vi "Periodic Tasks.vi"(8 "error in":errorcluster) -> ()   [LabVIEW 2019]
doc: "This VI runs in parallel to other tasks. It can contain as many user-defined periodic loops as you need. These can carry out PID or other sorts of timed response."
uses:
  <vilib>/Rock Robotics/WPI/DriverStation/WPI_DriverStationRobotMode2.ctl
  <vilib>/Rock Robotics/WPI/ThirdParty/Phoenix-LabVIEW/Motor Controller/Controls/CTRE_Phoenix_MotorControl_ControlMode.ctl
  <vilib>/Rock Robotics/WPI/Utilities/WPI_GetSetVariantRefNum.vi
  Robot Global Data.vi
  <vilib>/Rock Robotics/WPI/ThirdParty/Phoenix-LabVIEW/Pigeon IMU/CTRE_PigeonIMU_GetYPR.vi
  <vilib>/Rock Robotics/WPI/ThirdParty/Phoenix-LabVIEW/Motor Controller/Get/CTRE_Phoenix_MotorController_GetSelectedSensorData.vi
  <vilib>/Rock Robotics/Network Tables/NT Read Number.vi
  <vilib>/Rock Robotics/Network Tables/NT Write Number.vi
  <vilib>/addons/control/pid/pid.llb/PID (DBL).vi
  <vilib>/ptbypt/NI_PtbyPt.lvlib
  <vilib>/addons/control/pid/NI_PID_pid.lvlib
panel:
  out "Waveform Chart":dbl(graph)
  in  "RPM Range":dbl=120.0
  in  "Intake Speed 2":dbl(slide)=-1.0 min=-1.0 max=1.0 scale=-1.0..1.0
  in  "PID gains Shooter":T1={"proportional gain (Kc)"=0.0008, "integral time (Ti, min)"=0.0, "derivative time (Td, min)"=0.00015} {"derivative time (Td, min)" format="%.6f"; "integral time (Ti, min)" format="%.6f"; "proportional gain (Kc)" format="%.5f"}
  out "RPM Gauge":dbl
  in  "Shooter RPM":dbl=6000.0
  in  "Shooter RPM 3":dbl
  in  "Feeder Speed":dbl(slide)=1.0 min=-1.0 max=1.0 scale=-1.0..1.0
  in  "Conveyer Speed":dbl(slide)=-0.30612244897959184 min=-1.0 max=1.0 scale=-1.0..1.0
  in  "Intake Speed":dbl(slide)=1.0 min=-1.0 max=1.0 scale=-1.0..1.0
  in  "Feeder Speed 3":dbl(slide)=-1.0 min=-1.0 max=1.0 scale=-1.0..1.0
  in  "Conveyer Speed 3":dbl(slide)=0.16326530612244894 min=-1.0 max=1.0 scale=-1.0..1.0
  in  "Intake Speed 3":dbl(slide)=1.0 min=-1.0 max=1.0 scale=-1.0..1.0
  out "Turret Angle":dbl=90.48445184525423
  in  "PID gains Turret":T1={"proportional gain (Kc)"=0.01, "integral time (Ti, min)"=0.0, "derivative time (Td, min)"=0.0} {"derivative time (Td, min)" format="%.5f"; "integral time (Ti, min)" format="%.5f"; "proportional gain (Kc)" format="%.5f"}
  out "Go Slow?":bool
  in  "Z-axis rate modifier":dbl=0.7 format="%#_13g"
  in  "Slow Drive Speed %":dbl=0.75
  out "Robot Centric?":bool
  out "Sensor Loop Speed":u32=23
  in  "Sensor wait":u32=25
  out "Gyro Yaw Out":dbl=-111.95 format="%#_13g"
  out "Drive Loop Speed":u32=24
  in  "Drive wait":u32=25
  in  "Rot Pt Y":dbl format="%#_13g"
  in  "Rot Pt X":dbl format="%#_13g"
  out "Joystick Loop Speed":u32=24
  in  "Joystick wait":u32=25
  # "Intake"
  # "Shooter"
  # "Spinny wheel thing"
  # ".00050\n.000000\n.000100"
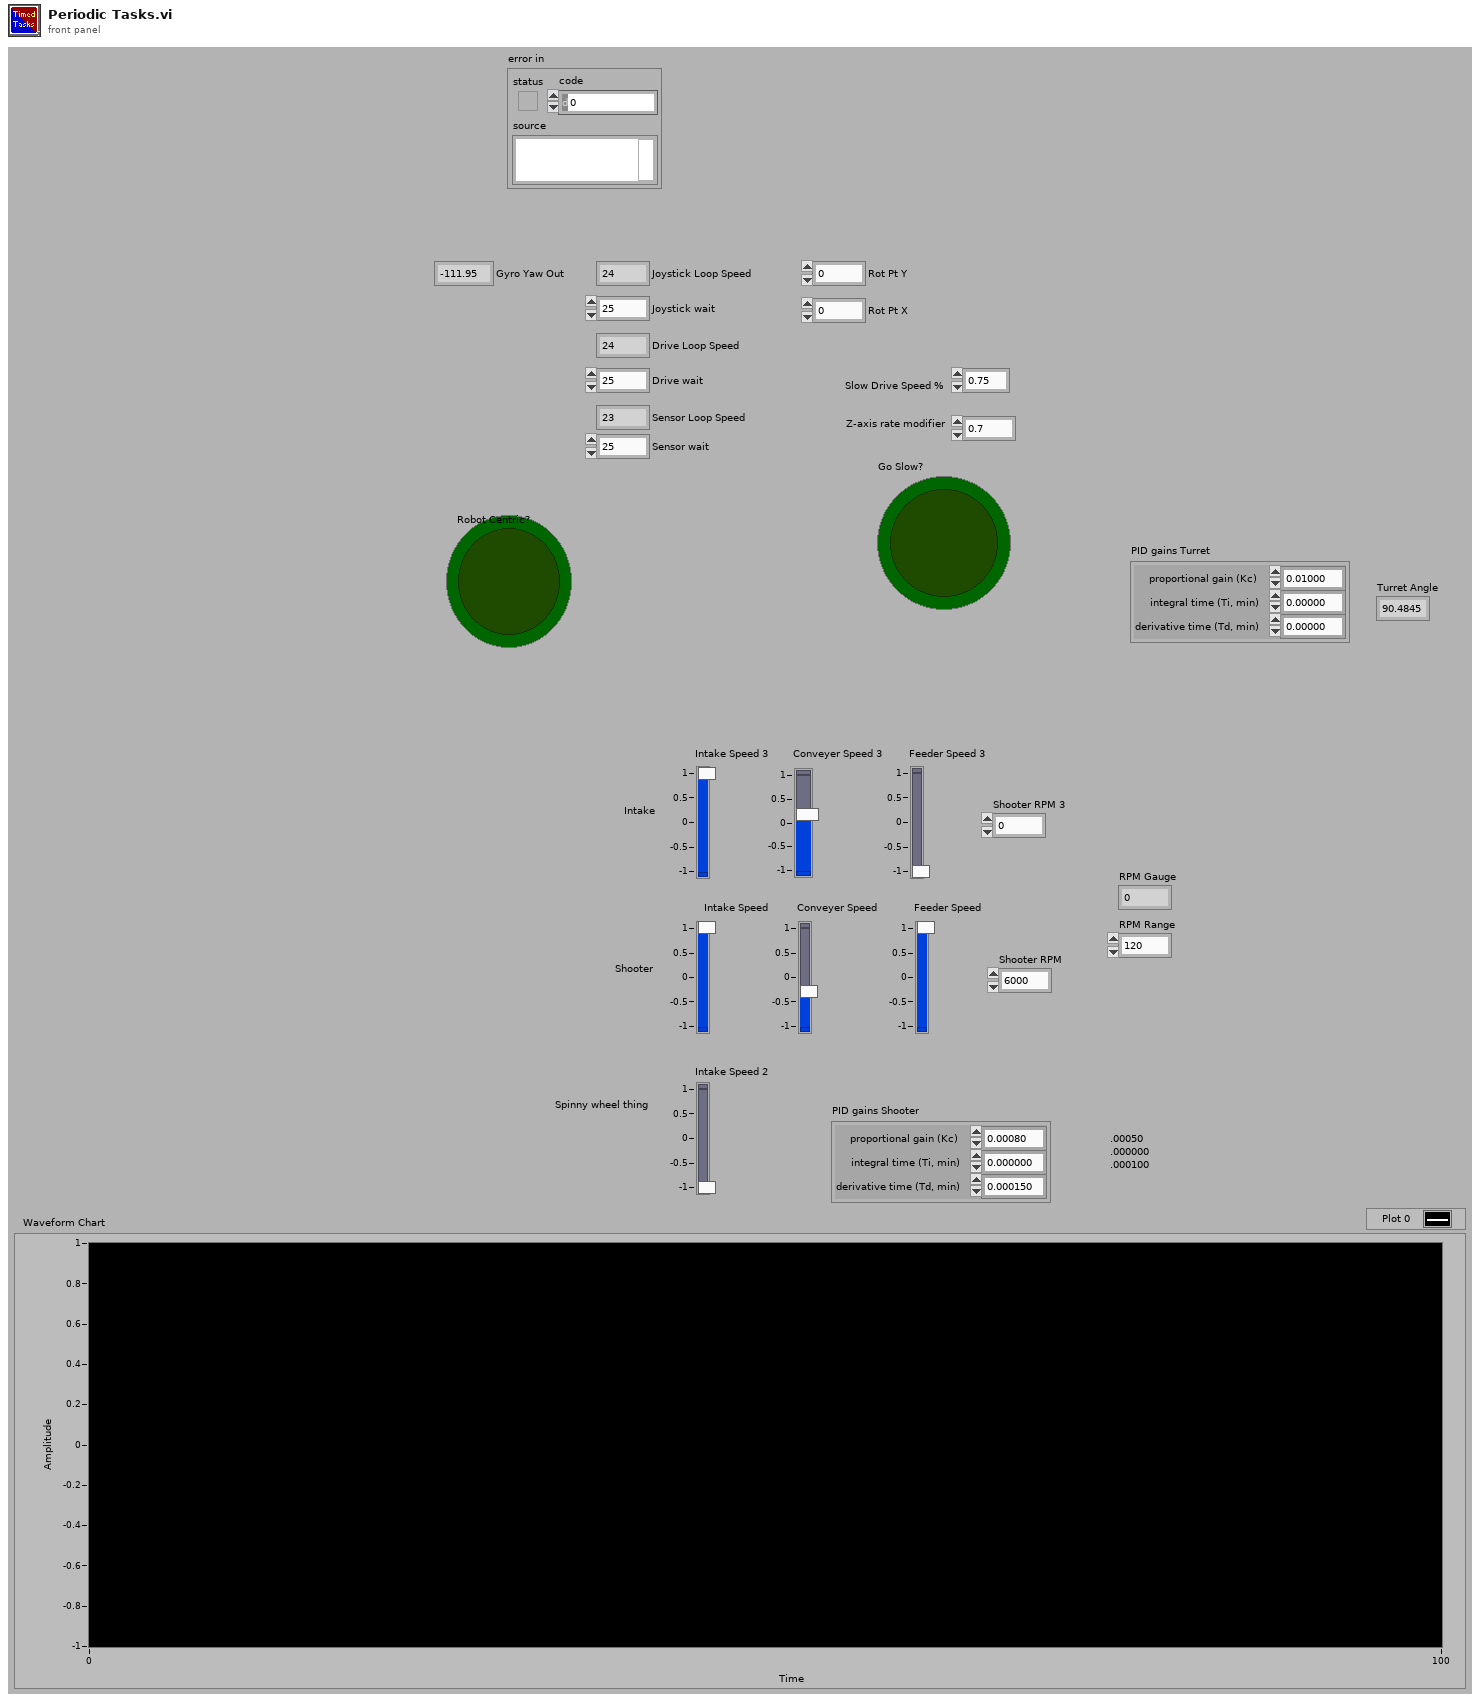
[diagram p1: front panel]
types:
  T1 = cluster{"proportional gain (Kc)":dbl, "integral time (Ti, min)":dbl, "derivative time (Td, min)":dbl}
  T2 = typedef "WPI_JoystickDevRef.ctl" = cluster{"Device":T3}
  T3 = typedef "WPI_JoystickDeviceEnum.ctl" = enum16{"USB 0", "USB 1", "USB 2", "USB 3", "USB 4", "USB 5"}
  T4 = typedef "WPI_DriverStationRobotMode2.ctl" = enum16{"Autonomous Disabled", "Autonomous Enabled", "Teleop Disabled", "Teleop Enabled", "Disconnected", "Finish", "Test Disabled", "Test Enabled", "Emergency Stopped"}
  T5 = typedef "CTRE_Phoenix_MotorControl_ControlMode.ctl" = u16
  T6 = typedef "CTRE_PigeonIMU_DeviceRef.ctl" = cluster{"DeviceStatus":errorcluster, "Device Number":u8, "Type":T7, "Device ID":u32, "Handle":u64, "UsageFrame":u32, "Library Path":path}
  T7 = typedef "CTRE_PigeonIMU_ConnectionType.ctl" = u32
  T8 = typedef "WPI_ServoDeviceRef.ctl" = cluster{"DeviceStatus":errorcluster, "PWM Channel":T9, "DeadBand":T10}
  T9 = typedef "FPGA_DIOPWMChannel.ctl" = enum8{"PWM 0", "PWM 1", "PWM 2", "PWM 3", "PWM 4", "PWM 5", "PWM 6", "PWM 7", "PWM 8", "PWM 9", "PWM MXP 0", "PWM MXP 1", "PWM MXP 2", "PWM MXP 3", "PWM MXP 4", "PWM MXP 5", "PWM MXP 6", "PWM MXP 7", "PWM MXP 8", "PWM MXP 9", "Invalid"}
  T10 = typedef "WPI_PWMDeadband.ctl" = cluster{"Name":string, "maxPositivePwm":i32, "minPositivePwm":i32, "centerPwm":i32, "maxNegativePwm":i32, "minNegativePwm":i32, "angularRange":u16}
  T11 = typedef "WPI_MotorControlDeviceRef.ctl" = cluster{"DeviceStatus":errorcluster, "Type":T12, "PWM":cluster{"PWM Channel":T9, "DeadBand":T10}, "CAN":cluster{"Device Number":u8, "SetOutput VI Ref":variant, "GetOutput VI Ref":variant, "Enable VI Ref":variant, "Disable VI Ref":variant, "Data":variant}, "Invert":bool, "DIO PWM":cluster{"PWM \"Enable\" Channel":T9, "DIOChannel":T13, "PWM Rate":dbl}}
  T12 = typedef "WPI_MotorControlType.ctl" = enum16{"PWM", "CAN", "DIO PWM"}
  T13 = typedef "FPGA_DIOChannel.ctl" = enum8{"DIO 0", "DIO 1", "DIO 2", "DIO 3", "DIO 4", "DIO 5", "DIO 6", "DIO 7", "DIO 8", "DIO 9", "DIO MXP 0", "DIO MXP 1", "DIO MXP 2", "DIO MXP 3", "DIO MXP 4", "DIO MXP 5", "DIO MXP 6", "DIO MXP 7", "DIO MXP 8", "DIO MXP 9", "DIO MXP 10", "DIO MXP 11", "DIO MXP 12", "DIO MXP 13", "DIO MXP 14", "DIO MXP 15", "SPI Port CS1", "SPI Port CS2", "SPI Port CS3", "SPI Port MISO", "SPI Port MOSI", "Invalid"}
  T14 = cluster{"Rollover":dbl, "Yaw":dbl, "Cont Yaw":dbl}
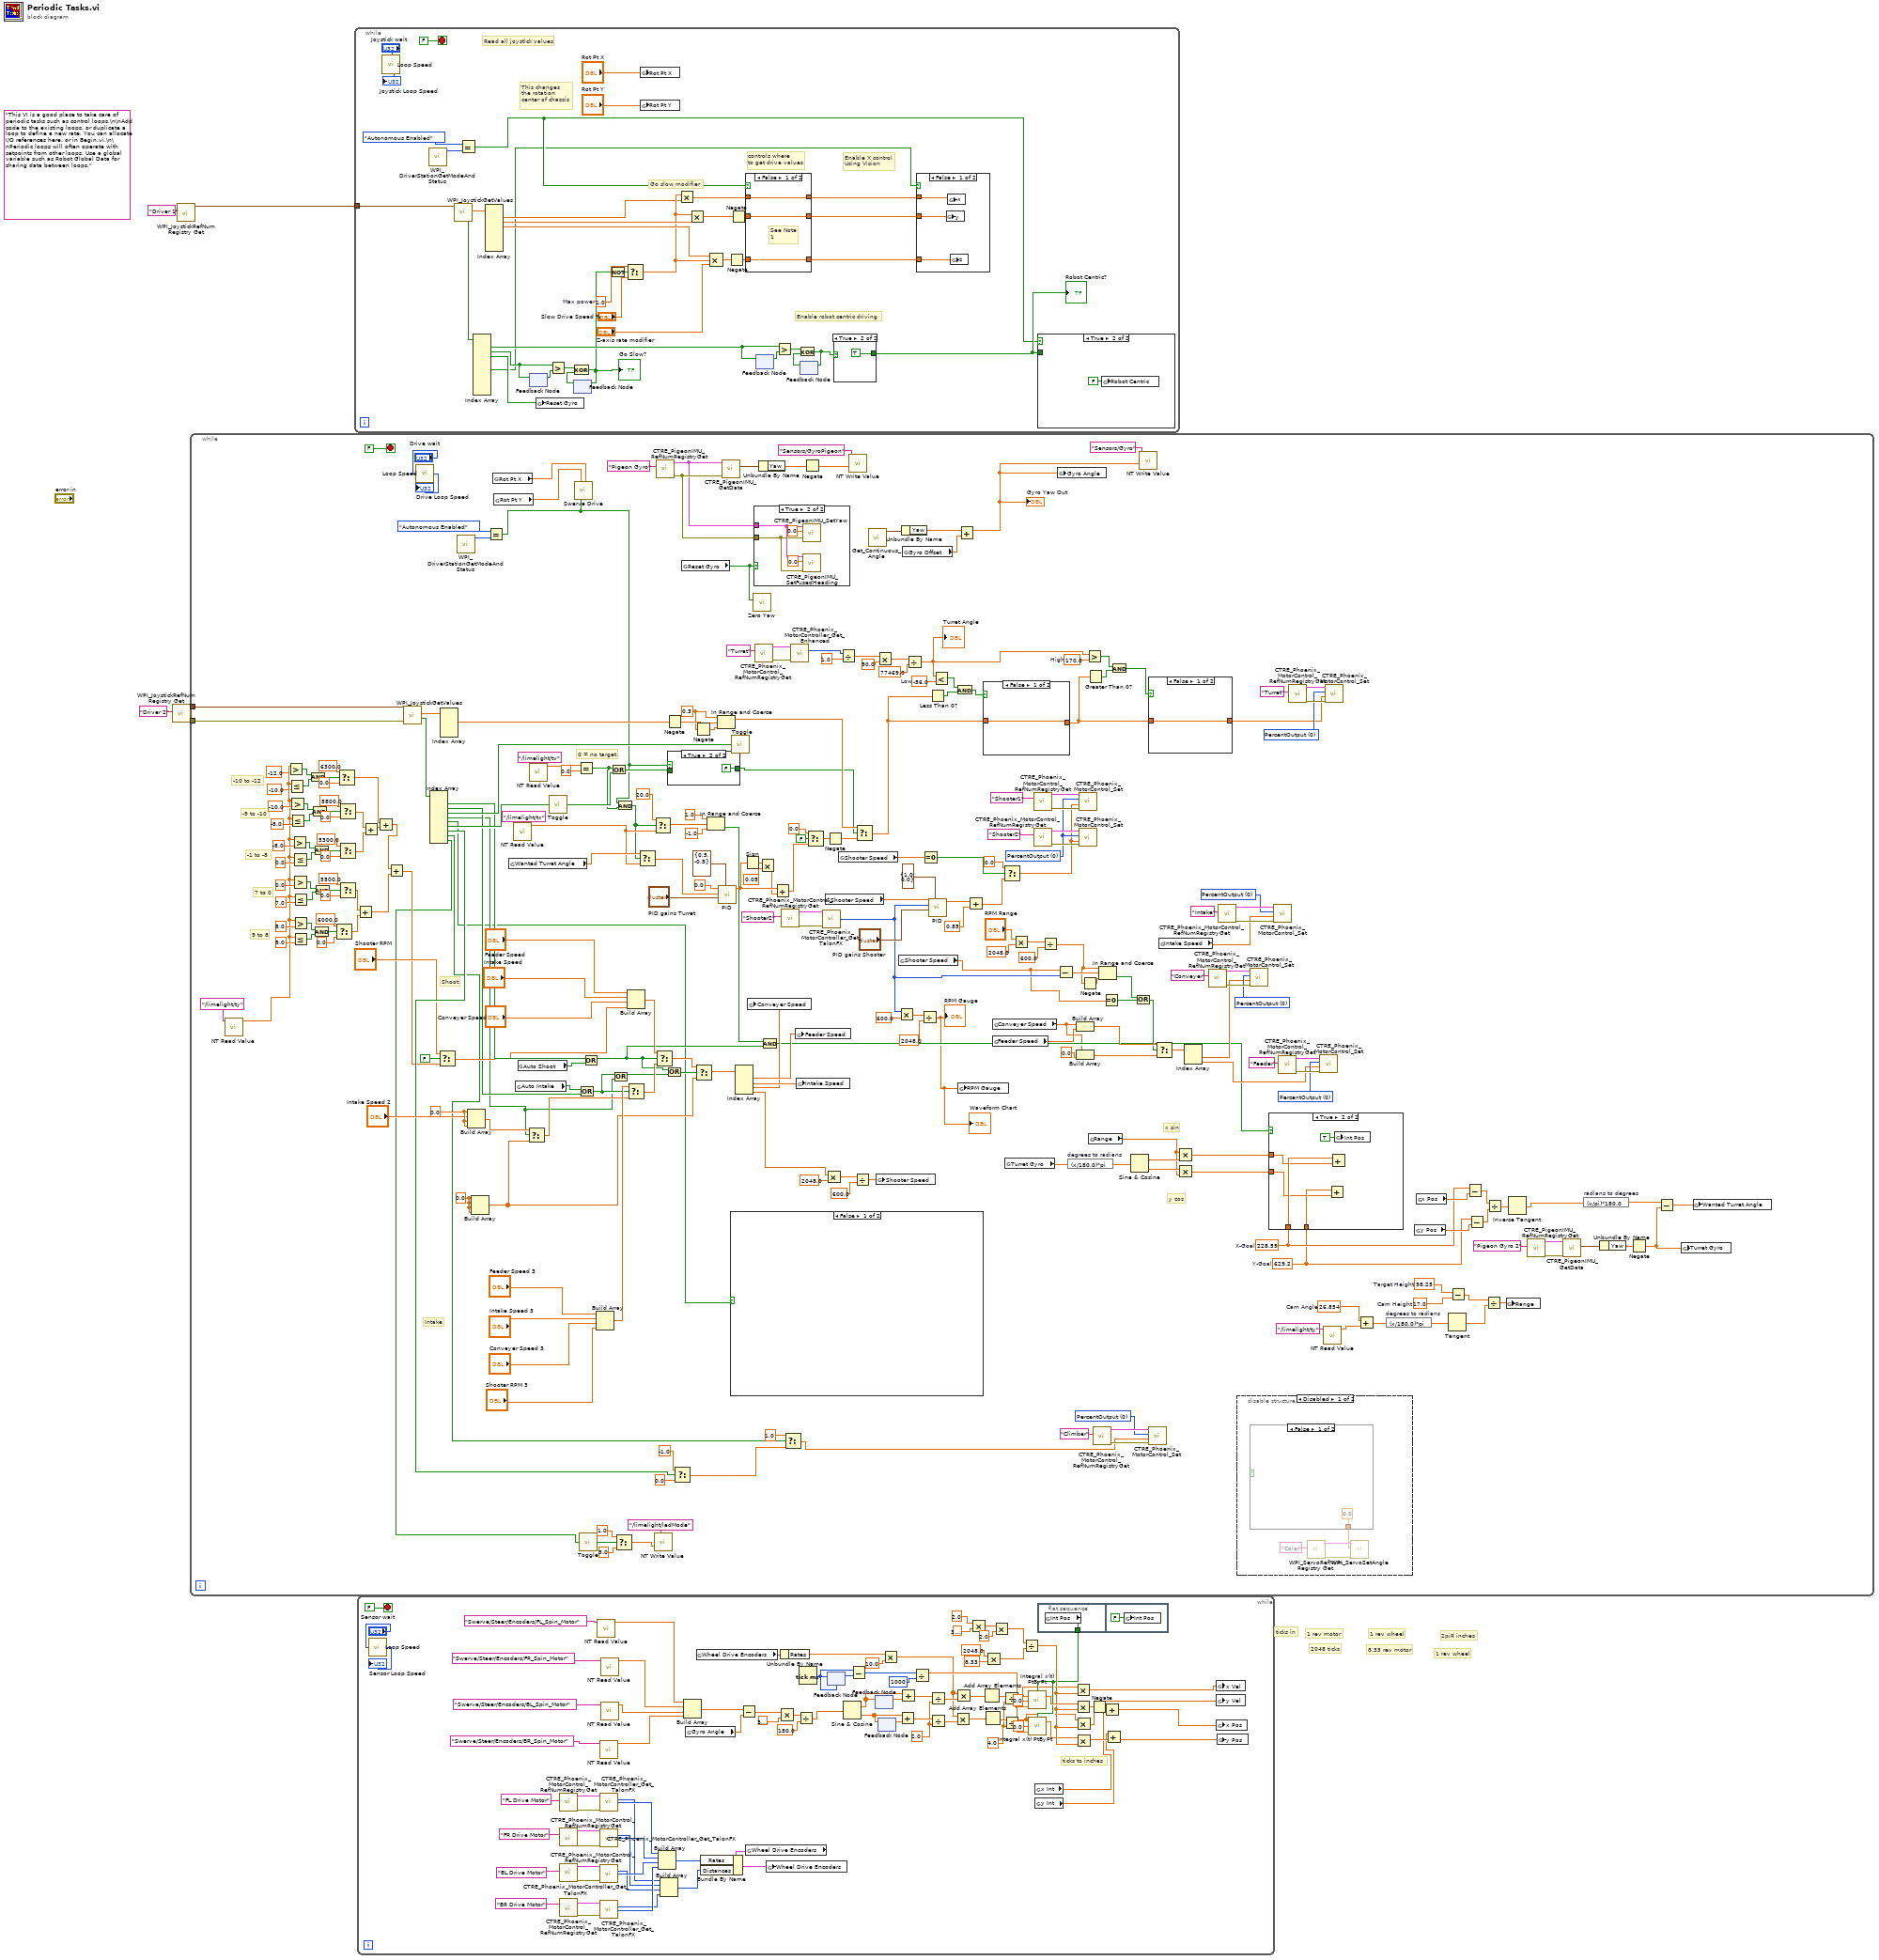
[diagram p0: block diagram]
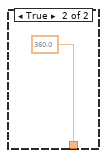
[diagram p2: hidden frame]
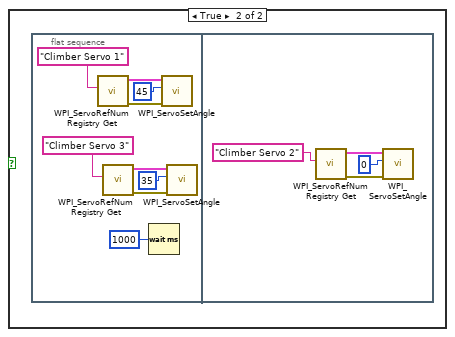
[diagram p6: hidden frame]
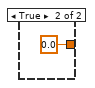
[diagram p7: hidden frame]
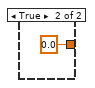
[diagram p8: hidden frame]
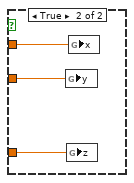
[diagram p10: hidden frame]
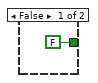
[diagram p11: hidden frame]
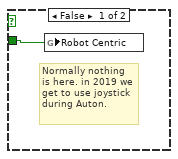
[diagram p12: hidden frame]
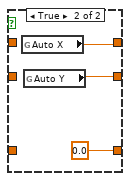
[diagram p13: hidden frame]
diagram:
  (unwired) "This VI is a good place to take care of periodic tasks such as control loops.\n\nAdd code to the existing loops, or duplicate a loop to define a new rate. You can allocate I/O references here, or in Begin.vi.\n\nPeriodic loops will often operate with setpoints from other loops. Use a global variable such as Robot Global Data for sharing data between loops."
  # "2piR inches"
  # "1 rev wheel"
  # "1 rev wheel"
  # "8.33 rev motor"
  # "1 rev motor"
  # "2048 ticks"
  # "ticks in"
  n1 = call <vilib>:"WPI_JoystickRefNum Registry Get.vi"("refnum name"="Driver 2") -> ("error out"=w2:errorcluster, "JoystickDevRef"=w1:T2)  [unwired: 9 in]
  n2 = call <vilib>:"WPI_JoystickRefNum Registry Get.vi"("refnum name"="Driver 1") -> ("JoystickDevRef"=w4:T2)  [unwired: 9 in, 1 out]
  n3 = while {
    tunnel: w2 -> [w233]
    tunnel: w1 -> [w232]
    stop <- FALSE stop-if-true
    w28 = T5 0 items=["PercentOutput"=0, "Position"=1, "Velocity"=2, "Current"=3, "Follower"=5, "MotionProfile"=6, "MotionMagic"=7, "MotionProfileArc"=10, "Disabled"=15] ("Control Mode")
    w109 = 26.854  # Cam Angle
    w112 = 17.0  # Cam Height
    w111 = 98.25  # Target Height
    w116 = 0.3 ("upper limit")
    w145 = T5 0 items=["PercentOutput"=0, "Position"=1, "Velocity"=2, "Current"=3, "Follower"=5, "MotionProfile"=6, "MotionMagic"=7, "MotionProfileArc"=10, "Disabled"=15] ("Control Mode")
    w149 = 228.59  # X-Goal
    w148 = 629.2  # Y-Goal
    w164 = 0.0 ("element")
    w203 = 0.0 ("element")
    w225 = T5 0 items=["PercentOutput"=0, "Position"=1, "Velocity"=2, "Current"=3, "Follower"=5, "MotionProfile"=6, "MotionMagic"=7, "MotionProfileArc"=10, "Disabled"=15] ("Control Mode")
    w223 = T5 0 items=["PercentOutput"=0, "Position"=1, "Velocity"=2, "Current"=3, "Follower"=5, "MotionProfile"=6, "MotionMagic"=7, "MotionProfileArc"=10, "Disabled"=15] ("Control Mode")
    w221 = T5 0 items=["PercentOutput"=0, "Position"=1, "Velocity"=2, "Current"=3, "Follower"=5, "MotionProfile"=6, "MotionMagic"=7, "MotionProfileArc"=10, "Disabled"=15] ("Control Mode")
    w251 = T5 0 items=["PercentOutput"=0, "Position"=1, "Velocity"=2, "Current"=3, "Follower"=5, "MotionProfile"=6, "MotionMagic"=7, "MotionProfileArc"=10, "Disabled"=15] ("Control Mode")
    w255 = 170.0  # High
    w263 = -56.0  # Low
    # "-10 to -12"
    # "-9 to -10"
    # "-1 to -8"
    # "7 to 0"
    # "9 to 8"
    # "y cos"
    # "x sin"
    # "0 = no target"
    # "Intake"
    # "Shoot"
    n4 = call-poly <vilib>:"NT Read Value.vi"("Name"="/limelight/ty") -> ("Numeric"=w8:dbl)  [unwired: 9 in, 1 out]
    n5 = Greater?(x=w8, y=-12.0) -> (0:w16:bool)
    n6 = Less Or Equal?(x=w8, y=-10.0) -> (x <= y?=w15:bool)
    n7 = Greater?(x=w8, y=-10.0) -> (0:w81:bool)
    n8 = Less Or Equal?(x=w8, y=-8.0) -> (x <= y?=w80:bool)
    n9 = Greater?(x=w8, y=-8.0) -> (0:w85:bool)
    n10 = Less Or Equal?(x=w8, y=0.0) -> (x <= y?=w84:bool)
    n11 = Greater?(x=w8, y=0.0) -> (0:w89:bool)
    n12 = Less Or Equal?(x=w8, y=7.0) -> (x <= y?=w88:bool)
    n13 = Greater?(x=w8, y=8.0) -> (0:w90:bool)
    n14 = Less Or Equal?(x=w8, y=9.0) -> (x <= y?=w91:bool)
    n15 = And(x=w16, y=w15) -> (x .and. y?=w14:bool)
    n16 = And(x=w81, y=w80) -> (x .and. y?=w79:bool)
    n17 = And(x=w85, y=w84) -> (x .and. y?=w78:bool)
    n18 = And(x=w90, y=w91) -> (x .and. y?=w76:bool)
    n19 = And(x=w89, y=w88) -> (x .and. y?=w77:bool)
    n20 = Select(t=6000.0, s=w76, f=0.0) -> (s? t:f=w66:dbl)
    n21 = Select(t=6300.0, s=w14, f=0.0) -> (s? t:f=w9:dbl)
    n22 = Select(t=5800.0, s=w79, f=0.0) -> (s? t:f=w65:dbl)
    n23 = Select(t=5300.0, s=w78, f=0.0) -> (s? t:f=w64:dbl)
    n24 = Select(t=5500.0, s=w77, f=0.0) -> (s? t:f=w67:dbl)
    n25 = Add(x=w67, y=w66) -> (x+y=w63:dbl)
    n26 = Add(x=w65, y=w64) -> (x+y=w11:dbl)
    n27 = Add(x=w9, y=w11) -> (x+y=w10:dbl)
    n28 = Add(x=w10, y=w63) -> (x+y=w62:dbl)
    n29 = call <vilib>:"WPI_JoystickGetValues.vi"("error in (no error)"=w233, "JoystickDevRef"=w232) -> ("Buttons"=w202:bool[], "Axes"=w249:dbl[])  [unwired: 5 in, 3 out]
    n30 = call "Loop Speed.vi"("milliseconds to wait"="Drive wait") -> ("Loop Speed"=→"Drive Loop Speed":u32)
    n31 = Index Array(array=w202) -> (element #1=w139:bool, element #2=w114:bool, element #3=w201:bool, element #4=w44:bool, element #5=w26:bool, element #6=w150:bool, element #7=w141:bool, element #8=w53:bool, element #9=w18:bool)  [unwired: 9 in]
    n32 = Select(t="Shooter RPM", s=FALSE, f=w62) -> (s? t:f=w124:dbl)
    n33 = Index Array(array=w249) -> (element #1=w241:dbl)  [unwired: 4 in, 3 out]
    n34 = call <vilib>:"WPI_DriverStationGetModeAndStatus.vi"() -> ("Robot Mode"=w283:T4)  [unwired: 10 in, 1 out]
    n35 = Build Array(w164, "Intake Speed 2", w164, w164) -> (w165:dbl[])
    n36 = Build Array(w203, w203, w203, w203) -> (w166:dbl[])
    n37 = Equal?(x=WPI_DriverStationRobotMode2."Autonomous Enabled", y=w283) -> (x = y?=w57:bool)
    n38 = global read "Robot Global Data.vi" "Rot Pt X"() -> (w274:dbl)
    n39 = global read "Robot Global Data.vi" "Rot Pt Y"() -> (w275:dbl)
    n40 = global read "Robot Global Data.vi" "Wanted Turret Angle"() -> (w152:dbl)
    n41 = call-poly <vilib>:"NT Read Value.vi"("Name"="/limelight/tx") -> ("Numeric"=w133:dbl)  [unwired: 9 in, 1 out]
    n42 = global read "Robot Global Data.vi" "Auto Intake"() -> (w113:bool)
    n43 = global read "Robot Global Data.vi" "Auto Shoot"() -> (w120:bool)
    n44 = Select(t=w165, s=w44, f=w166) -> (s? t:f=w167:dbl[])
    n45 = call-poly <vilib>:"NT Read Value.vi"("Name"="/limelight/tv") -> ("Numeric"=w238:dbl)  [unwired: 9 in, 1 out]
    n46 = call "Toggle.vi"("Input"=w150) -> ("Output"=w151:bool)
    n47 = call "Swerve Drive.vi"("Rot. Point X"=w274, "Auto Controls"=w57, "Rot. Point Y"=w275) -> ()  [unwired: 9 in]
    n48 = Equal?(x=w238, y=0.0) -> (x = y?=w60:bool)
    n49 = Or(x=w113, y=w114) -> (x .or. y?=w115:bool)
    n50 = call "Toggle.vi"("Input"=w18) -> ("Output"=w23:bool)
    n51 = Or(x=w139, y=w120) -> (x .or. y?=w121:bool)
    n52 = Build Array("Feeder Speed 3", "Intake Speed 3", "Conveyer Speed 3", "Shooter RPM 3") -> (w208:dbl[])
    n53 = Or(x=w60, y=w151) -> (x .or. y?=w59:bool)
    n54 = Or(x=w115, y=w44) -> (x .or. y?=w45:bool)
    n55 = Select(t=1.0, s=w23, f=3.0) -> (s? t:f=w19:dbl)
    n56 = And(x=w57, y=w60) -> (x .and. y?=w61:bool)
    n57 = Build Array("Feeder Speed", "Intake Speed", "Conveyer Speed", w124) -> (w212:dbl[])
    n58 = Select(t=w208, s=w115, f=w167) -> (s? t:f=w218:dbl[])
    n59 = Select(t=w152, s=w61, f=w133) -> (s? t:f=w159:dbl)
    n60 = Select(t=20.0, s=w61, f=w133) -> (s? t:f=w135:dbl)
    n61 = call-poly <vilib>:"NT Write Value.vi"("Numeric"=w19, "Name"="/limelight/ledMode") -> ()  [unwired: 9 in, 1 out]
    n62 = Select(t=w212, s=w121, f=w218) -> (s? t:f=w217:dbl[])
    n63 = call <vilib>:"CTRE_PigeonIMU_RefNumRegistryGet.vi"("refnum name"="Pigeon Gyro") -> ("error out"=w280:errorcluster, "PigeonIMUDevRef"=w279:T6)  [unwired: 9 in]
    n64 = Negate(x=w241) -> (-x=w119:dbl)
    n65 = Or(x=w121, y=w45) -> (x .or. y?=w216:bool)
    n66 = case shown="True" w57 {
      tunnel: w59 -> [w291 _]
      tunnel: [w291 FALSE] -> w58
      frame False {
      }
      frame True {
      }
    }
    n67 = Select(t=-1.0, s=w141, f=0.0) -> (s? t:f=w55:dbl)
    n68 = global read "Robot Global Data.vi" "Reset Gyro"() -> (w35:bool)
    n69 = Negate(x=w116) -> (-x=w117:dbl)
    n70 = Select(t=w217, s=w216, f=w166) -> (s? t:f=w207:dbl[])
    n71 = In Range and Coerce(upper limit=1.0, x=w135, lower limit=-1.0) -> (In Range?=w138:bool)  [unwired: 1 out]
    n72 = In Range and Coerce(upper limit=w116, x=w119, lower limit=w117) -> (coerced(x)=w118:dbl)  [unwired: 1 out]
    n73 = call-poly <vilib>:"PID.vi"("output range"=cluster{"output high":dbl, "output low":dbl} {"output high"=0.5, "output low"=-0.5}, "PID gains"="PID gains Turret", "process variable"=w159, "setpoint"=0.0) -> ("output"=w47:dbl)  [unwired: 6 in, 1 out]
    n74 = call-poly <vilib>:"CTRE_PigeonIMU_GetData.vi"("error in (no error)"=w280, "PigeonIMUDevRef"=w279) -> ("Yaw Pitch Roll"=w278:cluster{"Yaw":dbl, "Pitch":dbl, "Roll":dbl})  [unwired: 7 in, 2 out]
    n75 = case shown="False" w26 {
      frame False {
      }
      frame True {
        n76 = flat-sequence {
          frame #0 {
            n77 = call <vilib>:"WPI_ServoRefNum Registry Get.vi"("refnum name"="Climber Servo 1") -> ("error out"=w305:errorcluster, "ServoDeviceRef"=w304:T8)  [unwired: 9 in]
            n78 = call <vilib>:"WPI_ServoRefNum Registry Get.vi"("refnum name"="Climber Servo 3") -> ("error out"=w301:errorcluster, "ServoDeviceRef"=w300:T8)  [unwired: 9 in]
            n79 = Wait (ms)(milliseconds to wait=u32 1000) -> ()  [unwired: 1 out]
            n80 = call <vilib>:"WPI_ServoSetAngle.vi"("error in (no error)"=w305, "Angle"=45, "ServoDeviceRef"=w304) -> ()  [unwired: 7 in, 2 out]
            n81 = call <vilib>:"WPI_ServoSetAngle.vi"("error in (no error)"=w301, "Angle"=35, "ServoDeviceRef"=w300) -> ()  [unwired: 7 in, 2 out]
          }
          frame #1 {
            n82 = call <vilib>:"WPI_ServoRefNum Registry Get.vi"("refnum name"="Climber Servo 2") -> ("error out"=w310:errorcluster, "ServoDeviceRef"=w309:T8)  [unwired: 9 in]
            n83 = call <vilib>:"WPI_ServoSetAngle.vi"("error in (no error)"=w310, "Angle"=0, "ServoDeviceRef"=w309) -> ()  [unwired: 7 in, 2 out]
          }
        }
      }
    }
    n84 = call "Toggle.vi"("Input"=w201) -> ()  [unwired: 1 out]
    n85 = Index Array(array=w207) -> (element #1=w206:dbl, element #2=w205:dbl, element #3=w204:dbl, element #4=w172:dbl)  [unwired: 4 in]
    n86 = Sign(1:w47) -> (0:w49:dbl)
    n87 = global write "Robot Global Data.vi" "Conveyer Speed"(w204) -> ()
    n88 = call <vilib>:"Zero Yaw.vi"("Zero"=w35) -> ()  [unwired: 11 in]
    n89 = case shown="True" w35 {
      tunnel: w279 -> [_ w316]
      tunnel: w280 -> [_ w315]
      frame False {
      }
      frame True {
        n90 = call <vilib>:"CTRE_PigeonIMU_SetYaw.vi"("error in (no error)"=w315, "Value"=0.0, "PigeonIMUDevRef"=w316) -> ()  [unwired: 7 in, 2 out]
        n91 = call <vilib>:"CTRE_PigeonIMU_SetFusedHeading.vi"("error in (no error)"=w315, "Value"=0.0, "PigeonIMUDevRef 2"=w316) -> ()  [unwired: 7 in, 2 out]
      }
    }
    n92 = call <vilib>:"CTRE_Phoenix_MotorControl_RefNumRegistryGet.vi"("refnum name"="Turret") -> ("error out"=w264:errorcluster, "PhoenixMotorControlDevRef"=w265:T11)  [unwired: 9 in]
    n93 = Unbundle By Name(w278) -> ("Yaw"=w281:dbl)
    n94 = Multiply(x=w49, y=0.05) -> (x*y=w46:dbl)
    n95 = And(x=w138, y=w121) -> (x .and. y?=w140:bool)
    n96 = Add(x=w47, y=w46) -> (x+y=w50:dbl)
    n97 = call <vilib>:"CTRE_Phoenix_MotorControl_RefNumRegistryGet.vi"("refnum name"="Shooter2") -> ("error out"=w199:errorcluster, "PhoenixMotorControlDevRef"=w198:T11)  [unwired: 9 in]
    n98 = Select(t=1.0, s=w53, f=w55) -> (s? t:f=w56:dbl)
    n99 = call-poly <vilib>:"CTRE_Phoenix_MotorController_Get_Enhanced.vi"("PhoenixMotorControlDevRef"=w265, "error in"=w264) -> ("Position (Raw Sensor Units)"=w236:i32)  [unwired: 10 in, 3 out]
    n100 = global write "Robot Global Data.vi" "Feeder Speed"(w206) -> ()
    n101 = global write "Robot Global Data.vi" "Intake Speed"(w205) -> ()
    n102 = Negate(x=w281) -> (-x=w36:dbl)
    n103 = Select(t=0.0, s=FALSE, f=w50) -> (s? t:f=w234:dbl)
    n104 = call-poly <vilib>:"CTRE_Phoenix_MotorController_Get_TalonFX.vi"("PhoenixMotorControlDevRef"=w198, "error in"=w199) -> ("Velocity (Raw Sensor Units per 100 ms)"=w132:i32)  [unwired: 10 in, 3 out]
    n105 = global read "Robot Global Data.vi" "Shooter Speed"() -> (w182:dbl)
    n106 = Multiply(x=w172, y=2048.0) -> (x*y=w174:dbl)
    n107 = Negate(x=w234) -> (-x=w137:dbl)
    n108 = global read "Robot Global Data.vi" "Shooter Speed"() -> (w185:dbl)
    n109 = Divide(x=w236, y=1.0) -> (x/y=w270:dbl)
    n110 = call-poly <vilib>:"NT Write Value.vi"("Numeric"=w36, "Name"="Sensors/GyroPigeon") -> ()  [unwired: 9 in, 1 out]
    n111 = Divide(x=w174, y=600.0) -> (x/y=w171:dbl)
    n112 = Select(t=w118, s=w58, f=w137) -> (s? t:f=w240:dbl)
    n113 = call <vilib>:"Get_Continuous_Angle.vi"() -> ("Continuous Angle"=w39:T14)  [unwired: 11 in]
    n114 = Multiply(x=w270, y=90.0) -> (x*y=w268:dbl)
    n115 = global write "Robot Global Data.vi" "Shooter Speed"(w171) -> ()
    n116 = Multiply(x=w132, y=600.0) -> (x*y=w169:dbl)
    n117 = global read "Robot Global Data.vi" "Shooter Speed"() -> (w131:dbl)
    n118 = Unbundle By Name(w39) -> ("Yaw"=w38:dbl)
    n119 = global read "Robot Global Data.vi" "Gyro Offset"() -> (w24:dbl)
    n120 = Divide(x=w268, y=77469.0) -> (x/y=w235:dbl)
    "Turret Angle" <- w235
    n121 = Divide(x=w169, y=2048.0) -> (x/y=w17:dbl)
    "RPM Gauge" <- w17
    "Waveform Chart" <- w17
    n122 = Equal To 0?(x=w185) -> (x = 0?=w183:bool)
    n123 = call-poly <vilib>:"PID.vi"("output range"=cluster{"output high":dbl, "output low":dbl} {"output high"=1.0, "output low"=0.0}, "PID gains"="PID gains Shooter", "process variable"=w132, "setpoint"=w182) -> ("output"=w178:dbl)  [unwired: 6 in, 1 out]
    n124 = Less Than 0?(x=w240) -> (x < 0?=w261:bool)
    n125 = Less?(x=w235, y=w263) -> (x < y?=w262:bool)
    n126 = And(x=w262, y=w261) -> (x .and. y?=w260:bool)
    n127 = Add(x=w38, y=w24) -> (x+y=w25:dbl)
    "Gyro Yaw Out" <- w25
    n128 = global write "Robot Global Data.vi" "RPM Gauge"(w17) -> ()
    n129 = Add(x=w178, y=0.85) -> (x+y=w179:dbl)
    n130 = case shown="False" w260 {
      tunnel: [w313 0.0] -> w259
      tunnel: w240 -> [w313 _]
      frame False {
      }
      frame True {
      }
    }
    n131 = global read "Robot Global Data.vi" "Conveyer Speed"() -> (w52:dbl)
    n132 = global read "Robot Global Data.vi" "Feeder Speed"() -> (w194:dbl)
    n133 = Select(t=0.0, s=w183, f=w179) -> (s? t:f=w27:dbl)
    n134 = global read "Robot Global Data.vi" "Turret Gyro"() -> (w103:dbl)
    n135 = Multiply(x="RPM Range", y=2048.0) -> (x*y=w129:dbl)
    n136 = call <vilib>:"CTRE_Phoenix_MotorControl_RefNumRegistryGet.vi"("refnum name"="Shooter1") -> ("error out"=w31:errorcluster, "PhoenixMotorControlDevRef"=w32:T11)  [unwired: 9 in]
    n137 = call <vilib>:"CTRE_Phoenix_MotorControl_RefNumRegistryGet.vi"("refnum name"="Shooter2") -> ("error out"=w29:errorcluster, "PhoenixMotorControlDevRef"=w30:T11)  [unwired: 9 in]
    n138 = Divide(x=w129, y=600.0) -> (x/y=w127:dbl)
    n139 = Subtract(x=w131, y=w132) -> (x-y=w196:dbl)
    n140 = global write "Robot Global Data.vi" "Gyro Angle"(w25) -> ()
    n141 = expression code="(x/180.0)*pi" "degrees to radians"(w103) -> (w102:dbl)
    n142 = Build Array(w52, w194) -> (w193:dbl[])
    n143 = Build Array(w52, 0.0 ("element")) -> (w191:dbl[])
    n144 = call <vilib>:"CTRE_Phoenix_MotorControl_Set.vi"("error in (no error)"=w31, "Output"=w27, "Control Mode"=w28, "PhoenixMotorControlDevRef"=w32) -> ()  [unwired: 6 in, 2 out]
    n145 = call <vilib>:"CTRE_Phoenix_MotorControl_Set.vi"("error in (no error)"=w29, "Output"=w27, "Control Mode"=w28, "PhoenixMotorControlDevRef"=w30) -> ()  [unwired: 6 in, 2 out]
    n146 = Negate(x=w127) -> (-x=w195:dbl)
    n147 = Greater?(x=w235, y=w255) -> (0:w257:bool)
    n148 = Greater Than 0?(x=w259) -> (x > 0?=w258:bool)
    n149 = global read "Robot Global Data.vi" "Range"() -> (w98:dbl)
    n150 = call <vilib>:"CTRE_Phoenix_MotorControl_RefNumRegistryGet.vi"("refnum name"="Climber") -> ("error out"=w147:errorcluster, "PhoenixMotorControlDevRef"=w146:T11)  [unwired: 9 in]
    n151 = In Range and Coerce(upper limit=w127, x=w196, lower limit=w195) -> (In Range?=w187:bool)  [unwired: 1 out]
    n152 = Equal To 0?(x=w131) -> (x = 0?=w186:bool)
    n153 = And(x=w257, y=w258) -> (x .and. y?=w256:bool)
    n154 = Sine & Cosine(0:w102) -> (1:w99:dbl, 2:w100:dbl)
    n155 = Or(x=w187, y=w186) -> (x .or. y?=w176:bool)
    n156 = call-poly <vilib>:"NT Write Value.vi"("Numeric"=w25, "Name"="Sensors/Gyro") -> ()  [unwired: 9 in, 1 out]
    n157 = call <vilib>:"CTRE_Phoenix_MotorControl_Set.vi"("error in (no error)"=w147, "Output"=w56, "Control Mode"=w145, "PhoenixMotorControlDevRef"=w146) -> ()  [unwired: 6 in, 2 out]
    n158 = case shown="False" w256 {
      tunnel: w259 -> [w311 _]
      tunnel: [w311 0.0] -> w250
      frame False {
      }
      frame True {
      }
    }
    n159 = Select(t=w193, s=w176, f=w191) -> (s? t:f=w190:dbl[])
    n160 = global read "Robot Global Data.vi" "Intake Speed"() -> (w219:dbl)
    n161 = Multiply(x=w98, y=w99) -> (x*y=w96:dbl)
    n162 = Multiply(x=w100, y=w98) -> (x*y=w97:dbl)
    n163 = Index Array(array=w190) -> (element #1=w189:dbl, element #2=w188:dbl)  [unwired: 2 in]
    n164 = call <vilib>:"CTRE_Phoenix_MotorControl_RefNumRegistryGet.vi"("refnum name"="Conveyer") -> ("error out"=w229:errorcluster, "PhoenixMotorControlDevRef"=w228:T11)  [unwired: 9 in]
    n165 = call <vilib>:"CTRE_Phoenix_MotorControl_RefNumRegistryGet.vi"("refnum name"="Intake") -> ("error out"=w227:errorcluster, "PhoenixMotorControlDevRef"=w226:T11)  [unwired: 9 in]
    n166 = disable-structure shown="Disabled" {
      frame Disabled {
        n167 = case shown="False" {
          selector: _ -> [_ _]
          tunnel: [0.0 ("Target") 360.0 ("Target")] -> w285
          frame False {
          }
          frame True {
          }
        }
        n168 = call <vilib>:"WPI_ServoRefNum Registry Get.vi"("refnum name"="Color") -> ("error out"=w286:errorcluster, "ServoDeviceRef"=w287:T8)  [unwired: 9 in]
        n169 = call <vilib>:"WPI_ServoSetAngle.vi"("error in (no error)"=w286, "Angle"=w285, "ServoDeviceRef"=w287) -> ()  [unwired: 7 in, 2 out]
      }
      frame Enabled {
      }
    }
    n170 = call <vilib>:"CTRE_Phoenix_MotorControl_Set.vi"("error in (no error)"=w229, "Output"=w189, "Control Mode"=w223, "PhoenixMotorControlDevRef"=w228) -> ()  [unwired: 6 in, 2 out]
    n171 = case shown="True" w140 {
      tunnel: w149 -> [_ w297]
      tunnel: w148 -> [_ w296]
      tunnel: w97 -> [_ w294]
      tunnel: w96 -> [_ w293]
      frame False {
      }
      frame True {
        n172 = Add(x=w296, y=w294) -> ()  [unwired: 1 out]
        n173 = Add(x=w297, y=w293) -> ()  [unwired: 1 out]
        n174 = global write "Robot Global Data.vi" "Int Pos"(TRUE ("Int Pos")) -> ()
      }
    }
    n175 = call <vilib>:"CTRE_Phoenix_MotorControl_Set.vi"("error in (no error)"=w227, "Output"=w219, "Control Mode"=w221, "PhoenixMotorControlDevRef"=w226) -> ()  [unwired: 6 in, 2 out]
    n176 = call <vilib>:"CTRE_Phoenix_MotorControl_RefNumRegistryGet.vi"("refnum name"="Feeder") -> ("error out"=w231:errorcluster, "PhoenixMotorControlDevRef"=w230:T11)  [unwired: 9 in]
    n177 = call <vilib>:"CTRE_Phoenix_MotorControl_RefNumRegistryGet.vi"("refnum name"="Turret") -> ("error out"=w252:errorcluster, "PhoenixMotorControlDevRef"=w253:T11)  [unwired: 9 in]
    n178 = call <vilib>:"CTRE_Phoenix_MotorControl_Set.vi"("error in (no error)"=w231, "Output"=w188, "Control Mode"=w225, "PhoenixMotorControlDevRef"=w230) -> ()  [unwired: 6 in, 2 out]
    n179 = call-poly <vilib>:"NT Read Value.vi"("Name"="/limelight/ty") -> ("Numeric"=w108:dbl)  [unwired: 9 in, 1 out]
    n180 = call <vilib>:"CTRE_Phoenix_MotorControl_Set.vi"("error in (no error)"=w252, "Output"=w250, "Control Mode"=w251, "PhoenixMotorControlDevRef"=w253) -> ()  [unwired: 6 in, 2 out]
    n181 = Add(x=w109, y=w108) -> (x+y=w107:dbl)
    n182 = expression code="(x/180.0)*pi" "degrees to radians"(w107) -> (w106:dbl)
    n183 = global read "Robot Global Data.vi" "y Pos"() -> (w162:dbl)
    n184 = global read "Robot Global Data.vi" "x Pos"() -> (w161:dbl)
    n185 = Tangent(1:w106) -> (0:w105:dbl)
    n186 = Subtract(x=w111, y=w112) -> (x-y=w110:dbl)
    n187 = Subtract(x=w149, y=w161) -> (x-y=w42:dbl)
    n188 = Subtract(x=w148, y=w162) -> (x-y=w43:dbl)
    n189 = Divide(x=w110, y=w105) -> (x/y=w104:dbl)
    n190 = Divide(x=w42, y=w43) -> (x/y=w41:dbl)
    n191 = global write "Robot Global Data.vi" "Range"(w104) -> ()
    n192 = Inverse Tangent(1:w41) -> (0:w40:dbl)
    n193 = call <vilib>:"CTRE_PigeonIMU_RefNumRegistryGet.vi"("refnum name"="Pigeon Gyro 2") -> ("error out"=w156:errorcluster, "PigeonIMUDevRef"=w155:T6)  [unwired: 9 in]
    n194 = call-poly <vilib>:"CTRE_PigeonIMU_GetData.vi"("error in (no error)"=w156, "PigeonIMUDevRef"=w155) -> ("Yaw Pitch Roll"=w154:cluster{"Yaw":dbl, "Pitch":dbl, "Roll":dbl})  [unwired: 7 in, 2 out]
    n195 = expression code="(x/pi)*180.0" "radians to degrees"(w40) -> (w160:dbl)
    n196 = Unbundle By Name(w154) -> ("Yaw"=w157:dbl)
    n197 = Negate(x=w157) -> (-x=w101:dbl)
    n198 = Subtract(x=w160, y=w101) -> (x-y=w158:dbl)
    n199 = global write "Robot Global Data.vi" "Turret Gyro"(w101) -> ()
    n200 = global write "Robot Global Data.vi" "Wanted Turret Angle"(w158) -> ()
  }
  n201 = while {
    tunnel: w4 -> [w320]
    stop <- FALSE stop-if-true
    w337 = 1.0  # Max power
    # "controls where\nto get drive values"
    # "Enable X control\nUsing Vision"
    # "Enable robot centric driving"
    # "Go slow modifier"
    # "This changes\nthe rotation\ncenter of chassis"
    # "Read all joystick values"
    n202 = call "Loop Speed.vi"("milliseconds to wait"="Joystick wait") -> ("Loop Speed"=→"Joystick Loop Speed":u32)
    n203 = call <vilib>:"WPI_DriverStationGetModeAndStatus.vi"() -> ("Robot Mode"=w324:T4)  [unwired: 10 in, 1 out]
    n204 = call <vilib>:"WPI_JoystickGetValues.vi"("JoystickDevRef"=w320) -> ("Buttons"=w352:bool[], "Axes"=w353:dbl[])  [unwired: 6 in, 3 out]
    n205 = Equal?(x=WPI_DriverStationRobotMode2."Autonomous Enabled", y=w324) -> (x = y?=w322:bool)
    n206 = Index Array(array=w352) -> (element #1=w346:bool, element #2=w333:bool, element #3=w350:bool, element #6=w319:bool)  [unwired: 11 in, 7 out]
    n207 = Index Array(array=w353) -> (element #1=w325:dbl, element #2=w351:dbl, element #5=w341:dbl)  [unwired: 8 in, 5 out]
    n208 = feedback #1() -> (w336:bool)  [unwired: 1 in]
    n209 = feedback-in #1(w333) -> ()
    n210 = global write "Robot Global Data.vi" "Reset Gyro"(w350) -> ()
    n211 = Greater?(x=w333, y=w336) -> (0:w335:bool)
    n212 = feedback #2() -> (w334:bool)  [unwired: 1 in]
    n213 = Exclusive Or(1:w334, 2:w335) -> (0:w332:bool)
    "Go Slow?" <- w332
    n214 = feedback-in #2(w332) -> ()
    n215 = Not(x=w332) -> (.not. x?=w331:bool)
    n216 = Select(t=w337, s=w331, f="Slow Drive Speed %") -> (s? t:f=w329:dbl)
    n217 = global write "Robot Global Data.vi" "Rot Pt X"("Rot Pt X") -> ()
    n218 = global write "Robot Global Data.vi" "Rot Pt Y"("Rot Pt Y") -> ()
    n219 = Multiply(x=w329, y=w325) -> (x*y=w339:dbl)
    n220 = Multiply(x=w329, y=w351) -> (x*y=w338:dbl)
    n221 = Compound Arithmetic op=MULTIPLY(w341, w329, "Z-axis rate modifier") -> (w330:dbl)
    n222 = Negate(x=w330) -> (-x=w343:dbl)
    n223 = Negate(x=w338) -> (-x=w344:dbl)
    n224 = case shown="False" w322 {
      tunnel: w344 -> [w370 _]
      tunnel: w339 -> [w369 _]
      tunnel: w343 -> [w371 _]
      tunnel: [w369 w372] -> w327
      tunnel: [w370 w373] -> w321
      tunnel: [w371 0.0] -> w328
      frame False {
        # "See Note\n1"
      }
      frame True {
        n225 = global read "Robot Global Data.vi" "Auto X"() -> (w372:dbl)
        n226 = global read "Robot Global Data.vi" "Auto Y"() -> (w373:dbl)
      }
    }
    n227 = feedback #3() -> (w349:bool)  [unwired: 1 in]
    n228 = feedback-in #3(w346) -> ()
    n229 = Greater?(x=w346, y=w349) -> (0:w348:bool)
    n230 = feedback #4() -> (w347:bool)  [unwired: 1 in]
    n231 = Exclusive Or(1:w347, 2:w348) -> (0:w345:bool)
    n232 = feedback-in #4(w345) -> ()
    n233 = case shown="True" w345 {
      tunnel: [FALSE TRUE] -> w326
      frame False {
      }
      frame True {
      }
    }
    "Robot Centric?" <- w326
    n234 = case shown="False" w319 {
      tunnel: w327 -> [w359 w363]
      tunnel: w328 -> [w361 w364]
      tunnel: w321 -> [w360 w362]
      frame False {
        n235 = global write "Robot Global Data.vi" "y"(w360) -> ()
        n236 = global write "Robot Global Data.vi" "x"(w359) -> ()
        n237 = global write "Robot Global Data.vi" "z"(w361) -> ()
      }
      frame True {
        n238 = global write "Robot Global Data.vi" "y"(w362) -> ()
        n239 = global write "Robot Global Data.vi" "z"(w364) -> ()
        n240 = global write "Robot Global Data.vi" "x"(w363) -> ()
      }
    }
    n241 = case shown="True" w322 {
      tunnel: w326 -> [w367 _]
      frame False {
        # "Normally nothing\nis here. in 2019 we\nget to use joystick\nduring Auton."
        n242 = global write "Robot Global Data.vi" "Robot Centric"(w367) -> ()
      }
      frame True {
        n243 = global write "Robot Global Data.vi" "Robot Centric"(FALSE ("Robot Centric")) -> ()
      }
    }
  }
  n244 = while {
    stop <- FALSE stop-if-true
    w386 = 4.0 ("y")
    w448 = 2.0
    # "ticks to inches"
    n245 = call "Loop Speed.vi"("milliseconds to wait"="Sensor wait") -> ("Loop Speed"=→"Sensor Loop Speed":u32)
    n246 = call <vilib>:"CTRE_Phoenix_MotorControl_RefNumRegistryGet.vi"("refnum name"="FL Drive Motor") -> ("error out"=w421:errorcluster, "PhoenixMotorControlDevRef"=w422:T11)  [unwired: 9 in]
    n247 = call <vilib>:"CTRE_Phoenix_MotorControl_RefNumRegistryGet.vi"("refnum name"="FR Drive Motor") -> ("error out"=w419:errorcluster, "PhoenixMotorControlDevRef"=w420:T11)  [unwired: 9 in]
    n248 = call <vilib>:"CTRE_Phoenix_MotorControl_RefNumRegistryGet.vi"("refnum name"="BL Drive Motor") -> ("error out"=w417:errorcluster, "PhoenixMotorControlDevRef"=w418:T11)  [unwired: 9 in]
    n249 = call <vilib>:"CTRE_Phoenix_MotorControl_RefNumRegistryGet.vi"("refnum name"="BR Drive Motor") -> ("error out"=w415:errorcluster, "PhoenixMotorControlDevRef"=w416:T11)  [unwired: 9 in]
    n250 = call-poly <vilib>:"NT Read Value.vi"("Name"="Swerve/Steer/Encoders/FL_Spin_Motor") -> ("Numeric"=w459:dbl)  [unwired: 9 in, 1 out]
    n251 = call-poly <vilib>:"NT Read Value.vi"("Name"="Swerve/Steer/Encoders/BR_Spin_Motor") -> ("Numeric"=w456:dbl)  [unwired: 9 in, 1 out]
    n252 = call-poly <vilib>:"CTRE_Phoenix_MotorController_Get_TalonFX.vi"("PhoenixMotorControlDevRef"=w422, "error in"=w421) -> ("Position (Raw Sensor Units)"=w396:i32, "Velocity (Raw Sensor Units per 100 ms)"=w432:i32)  [unwired: 10 in, 2 out]
    n253 = call-poly <vilib>:"CTRE_Phoenix_MotorController_Get_TalonFX.vi"("PhoenixMotorControlDevRef"=w420, "error in"=w419) -> ("Position (Raw Sensor Units)"=w428:i32, "Velocity (Raw Sensor Units per 100 ms)"=w431:i32)  [unwired: 10 in, 2 out]
    n254 = call-poly <vilib>:"CTRE_Phoenix_MotorController_Get_TalonFX.vi"("PhoenixMotorControlDevRef"=w418, "error in"=w417) -> ("Position (Raw Sensor Units)"=w427:i32, "Velocity (Raw Sensor Units per 100 ms)"=w430:i32)  [unwired: 10 in, 2 out]
    n255 = call-poly <vilib>:"CTRE_Phoenix_MotorController_Get_TalonFX.vi"("PhoenixMotorControlDevRef"=w416, "error in"=w415) -> ("Position (Raw Sensor Units)"=w426:i32, "Velocity (Raw Sensor Units per 100 ms)"=w429:i32)  [unwired: 10 in, 2 out]
    n256 = call-poly <vilib>:"NT Read Value.vi"("Name"="Swerve/Steer/Encoders/FR_Spin_Motor") -> ("Numeric"=w458:dbl)  [unwired: 9 in, 1 out]
    n257 = call-poly <vilib>:"NT Read Value.vi"("Name"="Swerve/Steer/Encoders/BL_Spin_Motor") -> ("Numeric"=w457:dbl)  [unwired: 9 in, 1 out]
    n258 = Build Array(w432, w431, w430, w429) -> (w383:i32[])
    n259 = Build Array(w396, w428, w427, w426) -> (w423:i32[])
    n260 = Build Array(w459, w458, w457, w456) -> (w455:dbl[])
    n261 = global read "Robot Global Data.vi" "Gyro Angle"() -> (w375:dbl)
    n262 = global read "Robot Global Data.vi" "Wheel Drive Encoders"() -> (w434:cluster{"Rates":dbl[], "Distances":dbl[]})
    n263 = Subtract(x=w455, y=w375) -> (x-y=w380:dbl[])
    n264 = global read "Robot Global Data.vi" "Wheel Drive Encoders"() -> (w425:cluster{"Rates":dbl[], "Distances":dbl[]})
    n265 = Bundle By Name(cluster=w425, "Rates"=w383, "Distances"=w423) -> (w424:cluster{"Rates":dbl[], "Distances":dbl[]})
    n266 = global write "Robot Global Data.vi" "Wheel Drive Encoders"(w424) -> ()
    n267 = Multiply(x=w380, y=3.141592653589793) -> (x*y=w379:dbl[])
    n268 = Unbundle By Name(w434) -> ("Rates"=w433:dbl[])
    n269 = Divide(x=w379, y=180.0) -> (x/y=w378:dbl[])
    n270 = Tick Count (ms)() -> (millisecond timer value=w442:u32)
    n271 = feedback #5(w442) -> (w443:u32)
    n272 = feedback-in #5(w442) -> ()
    n273 = Sine & Cosine(0:w378) -> (1:w453:dbl[], 2:w451:dbl[])
    n274 = Subtract(x=w442, y=w443) -> (x-y=w441:u32)
    n275 = feedback #6() -> (w454:dbl[])  [unwired: 1 in]
    n276 = feedback-in #6(w453) -> ()
    n277 = feedback #7() -> (w452:dbl[])  [unwired: 1 in]
    n278 = feedback-in #7(w451) -> ()
    n279 = Multiply(x=w433, y=10.0) -> (x*y=w390:dbl[])
    n280 = Add(x=w451, y=w452) -> (x+y=w449:dbl[])
    n281 = Add(x=w453, y=w454) -> (x+y=w450:dbl[])
    n282 = Divide(x=w441, y=u32 1000) -> (x/y=w392:dbl)
    n283 = Divide(x=w450, y=w448) -> (x/y=w447:dbl[])
    n284 = Divide(x=w449, y=w448) -> (x/y=w446:dbl[])
    n285 = Multiply(x=w390, y=w446) -> (x*y=w444:dbl[])
    n286 = Multiply(x=w390, y=w447) -> (x*y=w445:dbl[])
    n287 = Multiply(x=2.0, y=3.141592653589793) -> (x*y=w404:dbl)
    n288 = Add Array Elements(numeric array=w445) -> (sum=w384:dbl)
    n289 = Add Array Elements(numeric array=w444) -> (sum=w439:dbl)
    n290 = Multiply(x=2048.0, y=8.33) -> (x*y=w395:dbl)
    n291 = Multiply(x=w404, y=2.0) -> (x*y=w402:dbl)
    n292 = Divide(x=w384, y=w386) -> (x/y=w387:dbl)
    n293 = Divide(x=w439, y=w386) -> (x/y=w388:dbl)
    n294 = Divide(x=w402, y=w395) -> (x/y=w401:dbl)
    n295 = call <vilib>:"Integral x(t) PtByPt.vi"("initialize"=w397, "dt"=w392, "initial condition"=0.0, "x"=w387) -> ("integral x(t)"=w440:dbl)  [unwired: 1 out]
    n296 = call <vilib>:"Integral x(t) PtByPt.vi"("initialize"=w397, "dt"=w392, "initial condition"=0.0, "x"=w388) -> ("integral x(t)"=w398:dbl)  [unwired: 1 out]
    n297 = global read "Robot Global Data.vi" "x Int"() -> (w400:dbl)
    n298 = global read "Robot Global Data.vi" "y Int"() -> (w399:dbl)
    n299 = flat-sequence {
      tunnel: [w465] -> w397
      frame #0 {
        n300 = global read "Robot Global Data.vi" "Int Pos"() -> (w465:bool)
      }
      frame #1 {
        n301 = global write "Robot Global Data.vi" "Int Pos"(FALSE ("Int Pos")) -> ()
      }
    }
    n302 = Multiply(x=w387, y=w401) -> (x*y=w435:dbl)
    n303 = Multiply(x=w440, y=w401) -> (x*y=w438:dbl)
    n304 = Multiply(x=w388, y=w401) -> (x*y=w436:dbl)
    n305 = Multiply(x=w398, y=w401) -> (x*y=w437:dbl)
    n306 = Negate(x=w438) -> (-x=w385:dbl)
    n307 = Add(x=w385, y=w400) -> (x+y=w382:dbl)
    n308 = Add(x=w399, y=w437) -> (x+y=w381:dbl)
    n309 = global write "Robot Global Data.vi" "x Vel"(w435) -> ()
    n310 = global write "Robot Global Data.vi" "y Vel"(w436) -> ()
    n311 = global write "Robot Global Data.vi" "x Pos"(w382) -> ()
    n312 = global write "Robot Global Data.vi" "y Pos"(w381) -> ()
  }
